vi "mtg - check time to update.vi"(8 "error in (no error)":errorcluster, 10 "unit time (s)":dbl=1.0) -> (0 "error out":errorcluster, 2 "get reading":bool, 3 "xscale offset":dbl)   [LabVIEW 2025]
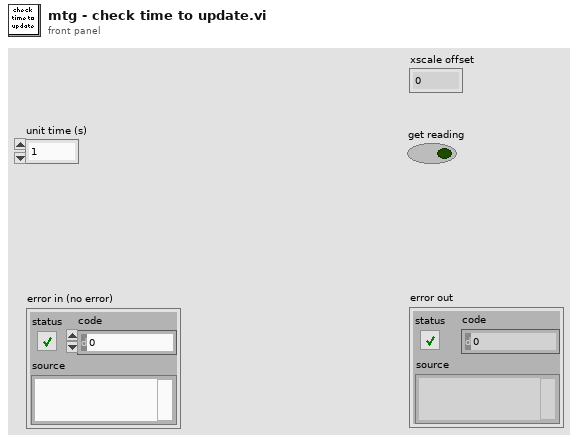
[diagram p1: front panel]
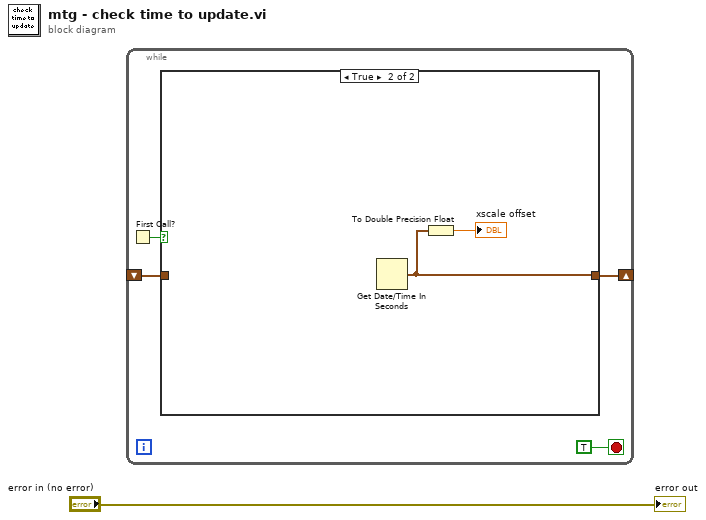
[diagram p0: block diagram]
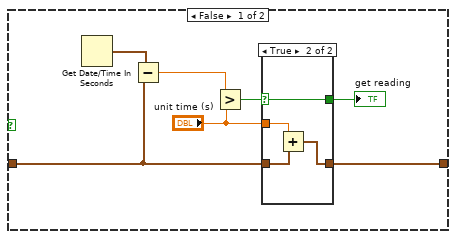
[diagram p2: hidden frame]
diagram:
  n1 = while {
    shift-right: [w5] -> _
    shift-left: _ -> [w4]
    stop <- TRUE stop-if-true
    n2 = First Call?() -> (First Call?: T/F=w2:bool)
    n3 = case shown="True" w2 {
      tunnel: [w11 w20] -> w5
      tunnel: w4 -> [w7 _]
      frame False {
        n4 = Get Date/Time In Seconds() -> (seconds since 1Jan1904=w6:timestamp)
        n5 = Subtract(x=w6, y=w7) -> (x-y=w8:dbl)
        n6 = Greater?(x=w8, y="unit time (s)") -> (0:w9:bool)
        n7 = case shown="True" w9 {
          selector: w9 -> [w14 w18]
          tunnel: w7 -> [w13 w17]
          tunnel: [w14 w18] -> w12
          tunnel: "unit time (s)" -> [_ w16]
          tunnel: [w13 w15] -> w11
          frame False {
          }
          frame True {
            n8 = Add(x=w16, y=w17) -> (x+y=w15:timestamp)
          }
        }
        "get reading" <- w12
      }
      frame True {
        n9 = Get Date/Time In Seconds() -> (seconds since 1Jan1904=w20:timestamp)
        n10 = To Double Precision Float(number=w20) -> (double precision float=→"xscale offset":dbl)
      }
    }
  }
  "error out" <- "error in (no error)"
